vi "GetClampMAXResultNames.vi"(7 "ProjectName":string="Prj", 10 "data":T1, 11 "ROI_Name":string="ROI1") -> (3 "ResultNames":string[](array[string]))   [LabVIEW 2019]
uses:
  Controls/Clamp MAX/Analysis_Clamp MAX_Result.ctl
  Controls/Clamp MAX/Analysis_Clamp MAX_Parameter.ctl
panel:
  in  "Analysis_ClampMAX_Result":T2 {"Clamp MAX Results"."Angle (Relative)" format="%.3f"; "Clamp MAX Results"."Angle (Absolute)" format="%.3f"; "Clamp MAX Results"."Distance (Real World)" format="%.3f"; "Clamp MAX Results"."Distance (Pixels)" format="%.3f"}
  out "error out":errorcluster
  in  "error in (no error)":errorcluster
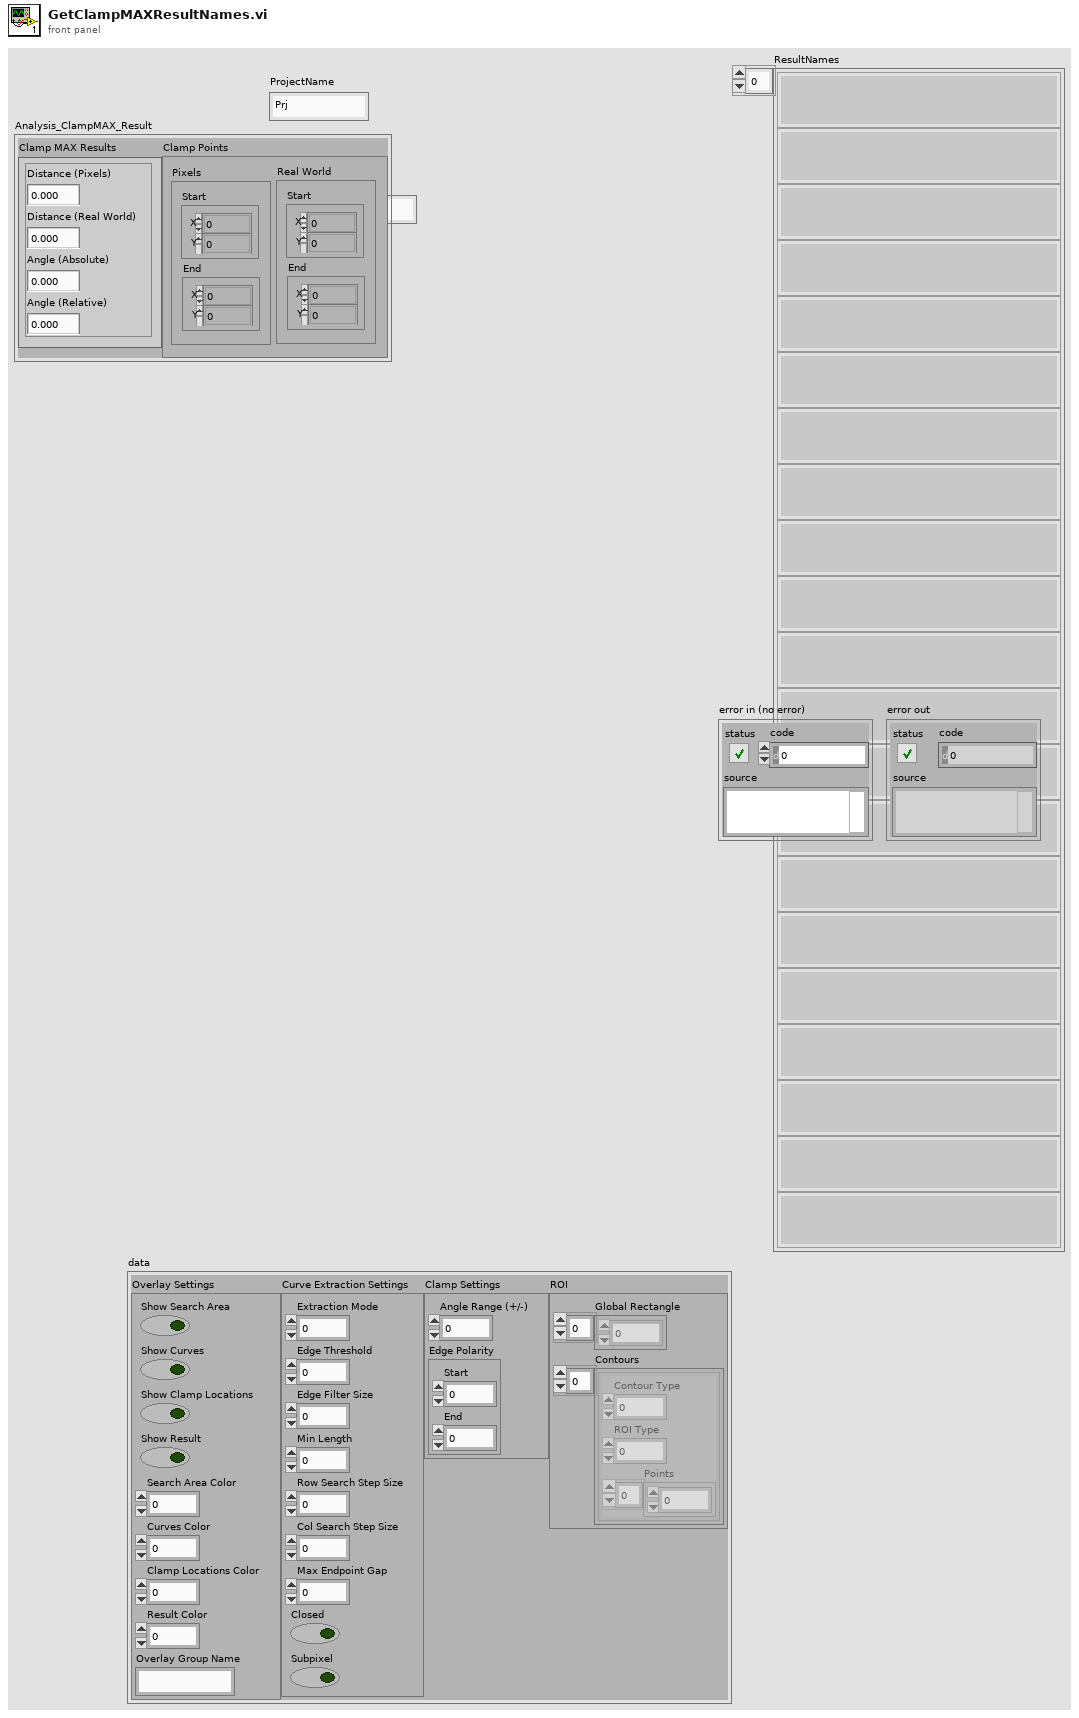
[diagram p1: front panel]
types:
  T1 = typedef "Analysis_Clamp MAX_Parameter.ctl" = cluster{"Overlay Settings":cluster{"Show Search Area":bool, "Show Curves":bool, "Show Clamp Locations":bool, "Show Result":bool, "Search Area Color":u32, "Curves Color":u32, "Clamp Locations Color":u32, "Result Color":u32, "Overlay Group Name":string}, "Curve Extraction Settings":cluster{"Extraction Mode":u32, "Edge Threshold":i32, "Edge Filter Size":u32, "Min Length":i32, "Row Search Step Size":i32, "Col Search Step Size":i32, "Max Endpoint Gap":i32, "Closed":bool, "Subpixel":bool}, "Clamp Settings":cluster{"Angle Range (+/-)":dbl, "Edge Polarity":cluster{"Start":u32, "End":u32}}, "ROI":cluster{"Global Rectangle":i32[], "Contours":cluster{"Contour Type":u32, "ROI Type":u32, "Points":i32[]}[]}}
  T2 = typedef "Analysis_Clamp MAX_Result.ctl" = cluster{"Clamp MAX Results":cluster{"Distance (Pixels)":dbl, "Distance (Real World)":dbl, "Angle (Absolute)":dbl, "Angle (Relative)":dbl}, "Clamp Points":cluster{"Pixels ":cluster{"Start":cluster{"X":dbl, "Y":dbl}, "End":cluster{"X":dbl, "Y":dbl}}, "Real World":cluster{"Start":cluster{"X":dbl, "Y":dbl}, "End":cluster{"X":dbl, "Y":dbl}}}}
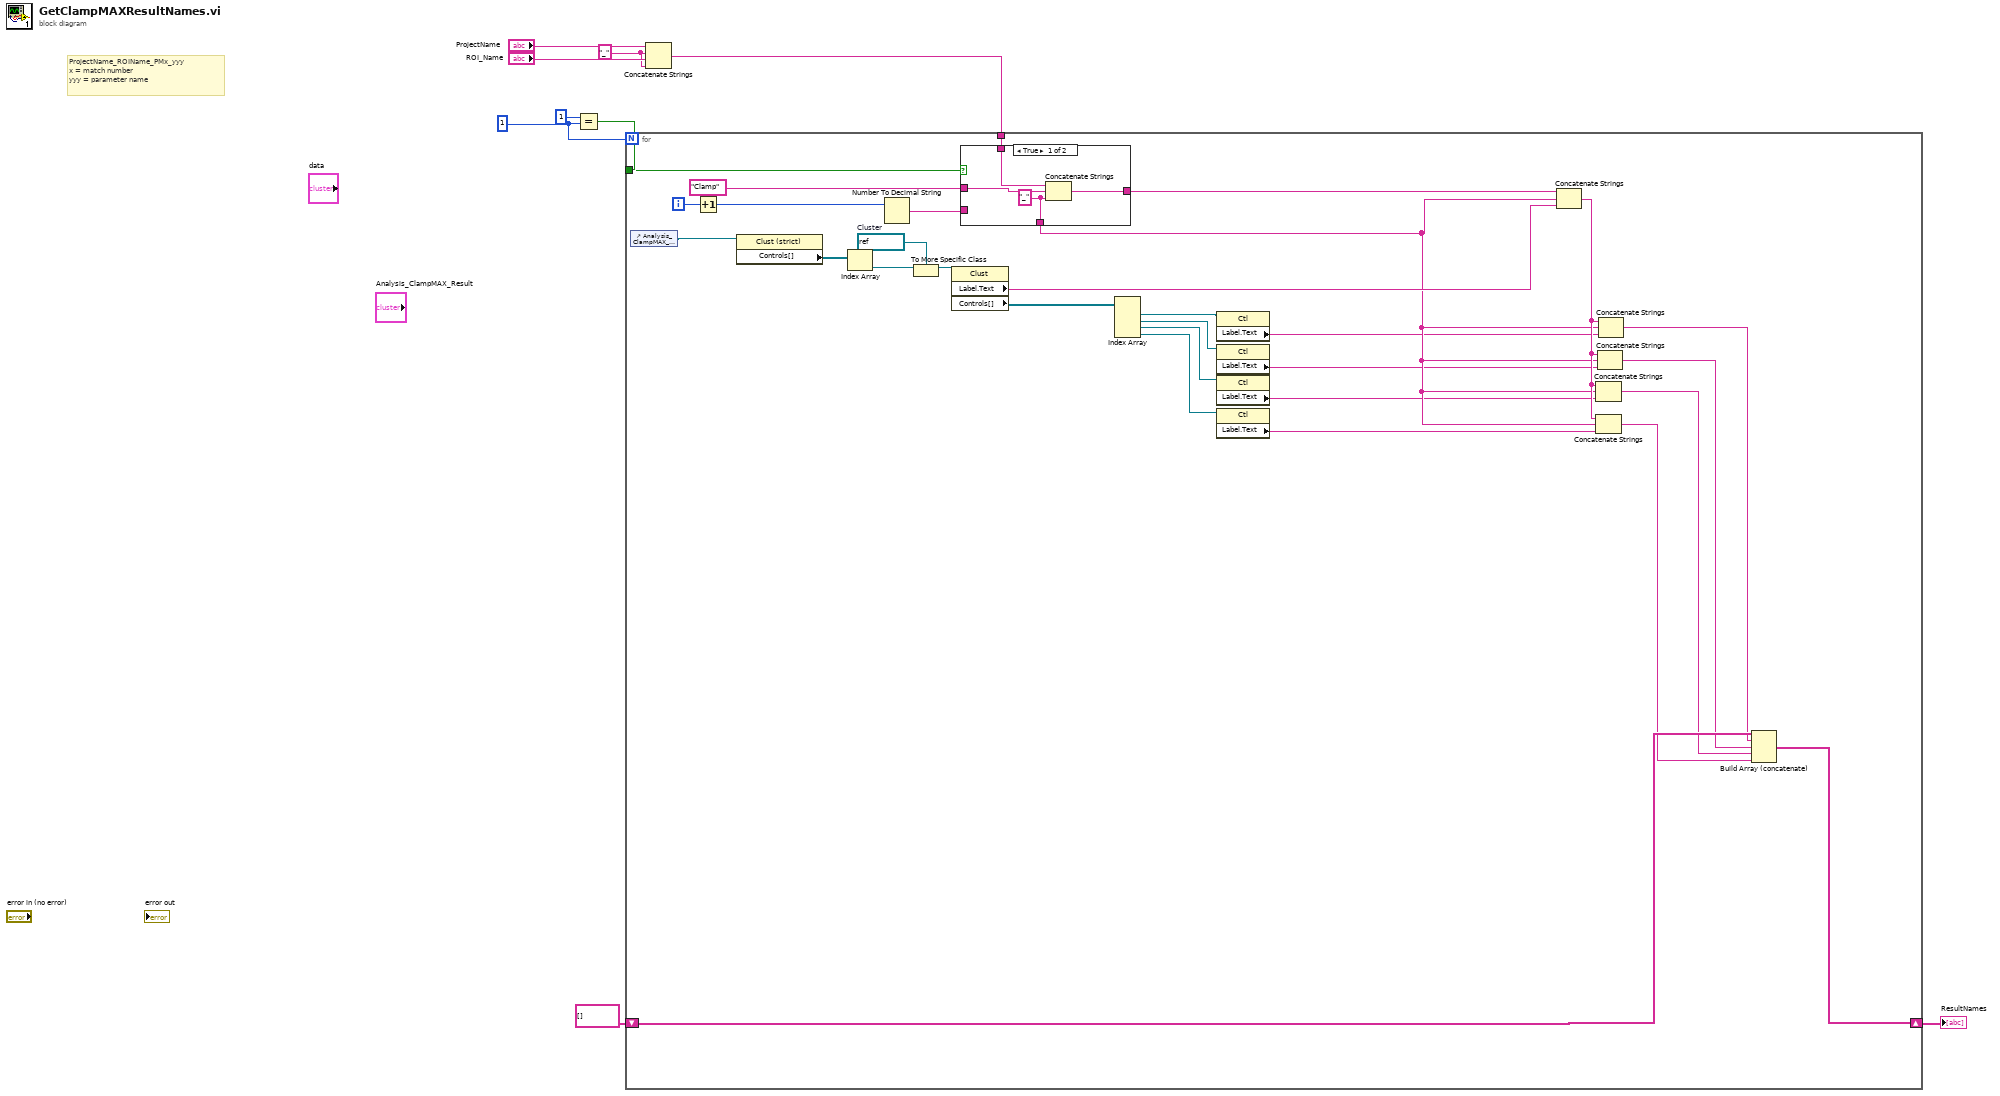
[diagram p0: block diagram]
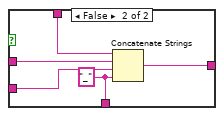
[diagram p2: hidden frame]
diagram:
  w1 = 1
  w6 = "_" ("string")
  # "ProjectName_ROIName_PMx_yyy\nx = match number\nyyy = parameter name"
  n1 = Equal?(x=1, y=w1) -> (x = y?=w2:bool)
  n2 = Concatenate Strings("ProjectName", w6, "ROI_Name", w6) -> (w5:string)
  n3 = for {
    N: w1 -> [_]
    tunnel: w5 -> [w37]
    shift-right: [w32] -> w3
    shift-left: string[] [] -> [w33]
    tunnel: w2 -> [w38]
    i -> [w34]
    w18 = refnum<vi> refnum  # Cluster
    n4 = control-ref of="Analysis_ClampMAX_Result"() -> (w29:refnum<vi>)
    n5 = Increment(x=w34) -> (x+1=w39:i32)
    n6 = property class="Clust (strict)"(reference=w29) -> ("Controls[]"=w20:refnum<vi>[])  [unwired: 1 in, 2 out]
    n7 = Index Array(array=w20) -> (element=w19:refnum<vi>)  [unwired: 1 in]
    n8 = Number To Decimal String(number=w39) -> (decimal integer string=w36:string)  [unwired: 1 in]
    n9 = To More Specific Class(target class=w18, reference=w19) -> (specific class reference=w17:refnum<vi>)  [unwired: 1 in, 1 out]
    n10 = property class="Clust"(reference=w17) -> ("Label.Text"=w15:string, "Controls[]"=w16:refnum<vi>[])  [unwired: 1 in, 2 out]
    n11 = case shown="True" w38 {
      tunnel: w37 -> [w43 w48]
      tunnel: w36 -> [_ w46]
      tunnel: [w42 w47] -> w30
      tunnel: "Clamp" ("string") -> [w41 w45]
      tunnel: [w40 w44] -> w14
      frame True {
        w40 = "_" ("string")
        n12 = Concatenate Strings(w43, w41, w40) -> (w42:string)
      }
      frame False {
        w44 = "_" ("string")
        n13 = Concatenate Strings(w48, w45, w46, w44) -> (w47:string)
      }
    }
    n14 = Index Array(array=w16) -> (element #1=w31:refnum<vi>, element #2=w28:refnum<vi>, element #3=w27:refnum<vi>, element #4=w26:refnum<vi>)  [unwired: 4 in]
    n15 = property class="Ctl"(reference=w31) -> ("Label.Text"=w13:string)  [unwired: 1 in, 2 out]
    n16 = property class="Ctl"(reference=w28) -> ("Label.Text"=w12:string)  [unwired: 1 in, 2 out]
    n17 = property class="Ctl"(reference=w27) -> ("Label.Text"=w11:string)  [unwired: 1 in, 2 out]
    n18 = property class="Ctl"(reference=w26) -> ("Label.Text"=w10:string)  [unwired: 1 in, 2 out]
    n19 = Concatenate Strings(w30, w14, w15) -> (w24:string)
    n20 = Concatenate Strings(w24, w14, w11) -> (w22:string)
    n21 = Concatenate Strings(w24, w14, w10) -> (w21:string)
    n22 = Concatenate Strings(w24, w14, w12) -> (w23:string)
    n23 = Concatenate Strings(w24, w14, w13) -> (w25:string)
    n24 = Build Array (concatenate)(w33, w25, w23, w22, w21) -> (w32:string[])
  }
  "ResultNames" <- w3
